vi "slope.vi"() -> ()   [LabVIEW 2011]
uses:
  <vilib>/Analysis/NI_AALPro.lvlib
panel:
  out "intercept":dbl
  out "slope":dbl
  out "Best Linear Fit":dbl[](array[numeric])
  in  "XY Graph":cluster{dbl[], dbl[]}(graph)
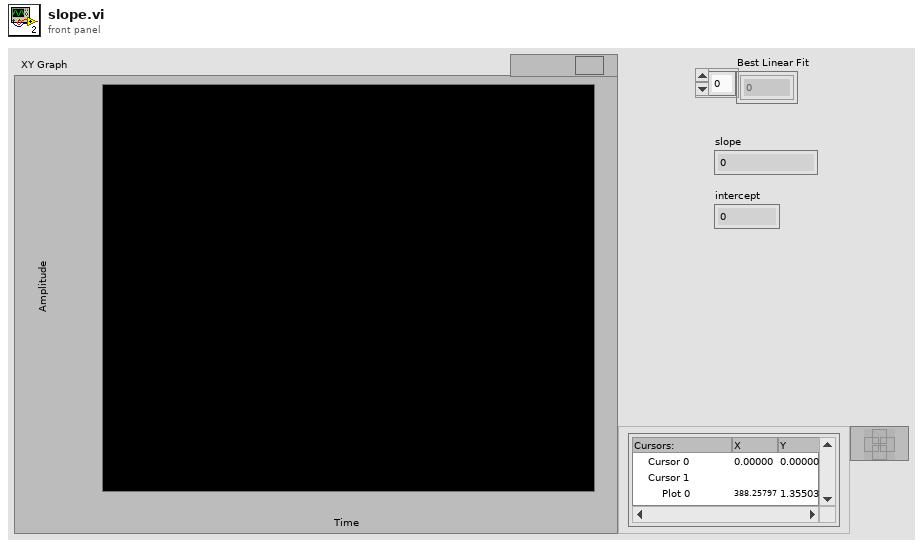
[diagram p1: front panel]
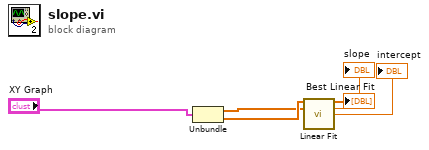
[diagram p0: block diagram]
diagram:
  n1 = Unbundle("XY Graph") -> (w1:dbl[], w2:dbl[])
  n2 = call <vilib>:"Linear Fit.vi"("Y"=w2, "X"=w1) -> ("Best Linear Fit"=→"Best Linear Fit":dbl[], "slope"=→"slope":dbl, "intercept"=→"intercept":dbl)  [unwired: 9 in, 2 out]
